vi "Gear Aiming PID.vi"(6 "PID gains":T1={"proportional gain (Kc)"=0.019, "integral time (Ti, min)"=0.0, "derivative time (Td, min)"=0.0} {"derivative time (Td, min)" format="%.3f"; "integral time (Ti, min)" format="%.3f"; "proportional gain (Kc)" format="%.3f"}, 9 "D":dbl, 10 "I":dbl, 11 "P":dbl) -> (3 "output":dbl)   [LabVIEW 2016]
uses:
  <vilib>/Rock Robotics/Network Tables/NT Read Number.vi
  Robot Global Data.vi
  <vilib>/addons/control/pid/pid.llb/PID (DBL).vi
  <vilib>/addons/control/pid/NI_PID_pid.lvlib
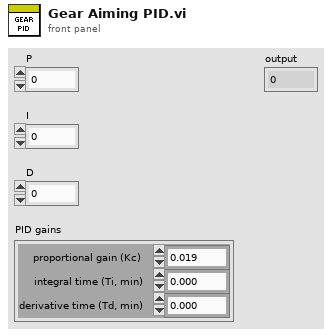
[diagram p1: front panel]
types:
  T1 = cluster{"proportional gain (Kc)":dbl, "integral time (Ti, min)":dbl, "derivative time (Td, min)":dbl}
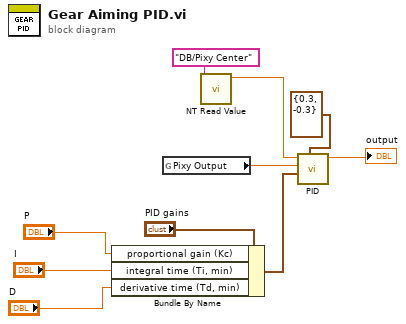
[diagram p0: block diagram]
diagram:
  n1 = Bundle By Name(cluster="PID gains", "proportional gain (Kc)"="P", "integral time (Ti, min)"="I", "derivative time (Td, min)"="D") -> (w6:T1)
  n2 = global read "Robot Global Data.vi" "Pixy Output"() -> (w5:dbl)
  n3 = call-poly <vilib>:"NT Read Value.vi"("Name"="DB/Pixy Center") -> ("Numeric"=w1:dbl)  [unwired: 9 in, 1 out]
  n4 = call-poly <vilib>:"PID.vi"("output range"=cluster{"output high":dbl, "output low":dbl} {"output high"=0.3, "output low"=-0.3}, "PID gains"=w6, "process variable"=w5, "setpoint"=w1) -> ("output"=→"output":dbl)  [unwired: 6 in, 1 out]
